vi "Global Lookup.vi"(8 "error in (no error)":errorcluster) -> (0 "error out":errorcluster, 3 "Global Lookup":refnum<data-value>)   [LabVIEW 2014, in "LVCOOOP Tests.lvlib"]
uses:
  LVCOOOP Tests.lvlib
  LVCOOOP/Lookup API/Providers/Default Lookup/Default Lookup.lvclass
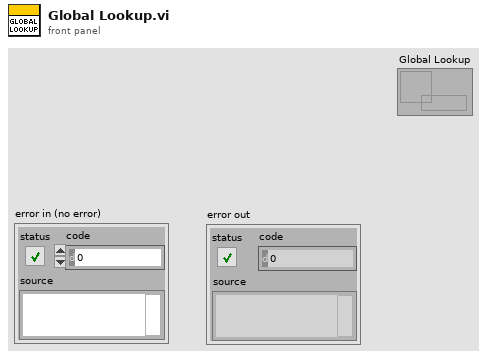
[diagram p1: front panel]
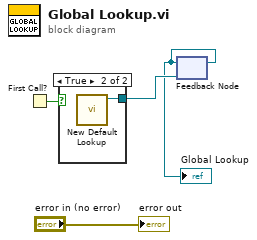
[diagram p0: block diagram]
diagram:
  n1 = First Call?() -> (First Call?: T/F=w2:bool)
  n2 = case shown="True" w2 {
    tunnel: [_ w5] -> w4
    frame False {
    }
    frame True {
      n3 = call "New Default Lookup.vi"() -> ("New Default Lookup"=w5:refnum<data-value>)  [unwired: 10 in, 1 out]
    }
  }
  n4 = feedback #1(w4) -> (w3:refnum<data-value>)
  "Global Lookup" <- w3
  n5 = feedback-in #1(w3) -> ()
  "error out" <- "error in (no error)"
